vi "CAMERATEST3.vi"() -> ()   [LabVIEW 2016, in "Test2.lvrbt"]
uses:
  Test2.lvrbt
  <vilib>/NXT/Block Support/NXT_InputPort.ctl
  <vilib>/NXT/Subs/ColorSensorColors.ctl
  <vilib>/NXT/Hardware/Plugins/Tetrix DC Motor/TetrixDCMotorAddress.ctl
  <vilib>/NXT/Hardware/Plugins/Tetrix 180 deg Servo/Tetrix180ServoAddress.ctl
  <vilib>/NXT/NXTIO Xnodes/NXTIONodeSubVIs/TETRIX IO Move Servos.vi
  <vilib>/NXT/Dual Mode Library/Waits/Wait_Num.vi
  <vilib>/NXT/NXTIO Xnodes/NXTIONodeSubVIs/TETRIX IO Move DC Motors.vi
  <vilib>/NXT/Dual Mode Library/Waits/Wait_EV3_Color_Color.vi
  <vilib>/NXT/NXTIO Xnodes/NXTIONodeSubVIs/TETRIX IO Stop DC Motors.vi
  <vilib>/NXT/Dual Mode Library/Sound/Tone.vi
  <vilib>/NXT/Dual Mode Library/Sound/StopSound.vi
  <vilib>/NXT/NXTIO Xnodes/AddressXNode/NXTIOAddress.xnode
  <vilib>/NXT/Subs/LVHSConnector.ctl
  <vilib>/NXT/NXTIO Xnodes/NXTIOXNode/NXTIO.xnode
  <vilib>/NXT/LegoClasses/BrickReference/BrickReference.lvclass
panel:
  out "Power":bool
  out "X Upper Left":u8
  out "X Lower Right":u8
  out "Y Lower Right":u8
  out "Y Upper Left":u8
  out "Count":u8
  out "Color":u8
  in  "Cluster":T1 {"Tracking Mode" items=["Disable Tracking", "Get First Object", "Get n th Object", "Enable Tracking", "Sort Objects  by size", "Sort Objects  by Colors", "Illumination on ", "Illumination Off", "Write Colormap", "Read Colormap", "Line tracking mode", "Object Tracking mode"]}
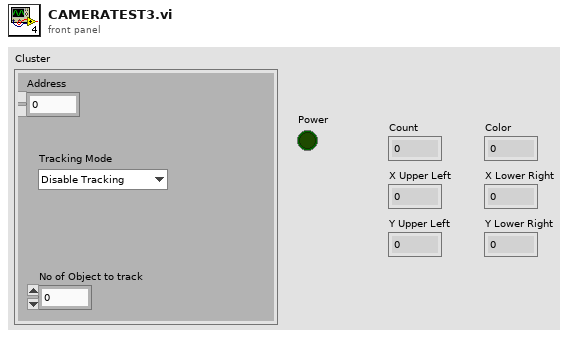
[diagram p1: front panel]
types:
  T1 = cluster{"Address":dbl, "No of Object to track":dbl, "Tracking Mode":u8}
  T2 = typedef "NXT_InputPort.ctl" = u32
  T3 = typedef "ColorSensorColors.ctl" = enum16{"No Color", "Black", "Blue", "Green", "Yellow", "Red", "White", "Brown"}
  T4 = cluster{"Tracking Mode":u8, "Object Number to Track":u8, "Address":u8}
  T5 = typedef "Tetrix180ServoAddress.ctl" = i32
  T6 = cluster{"Tetrix180Servo":T5, "Tetrix180Servo":T5, "Tetrix180Servo":T5, "Tetrix180Servo":T5, "Tetrix180Servo":T5, "Tetrix180Servo":T5}
  T7 = typedef "TetrixDCMotorAddress.ctl" = i32
  T8 = typedef "LVHSConnector.ctl" = refnum<class "BrickReference.lvclass">
  T9 = cluster{"TetrixDCMotor":T7, "TetrixDCMotor 2":T7}
  T10 = cluster{"Total Tracked Objects":u8, "Color":u8, "X Upper Left":u8, "Y Upper Left":u8, "X Lower Right":u8, "Y Lower Right":u8, "Status (boolean)":bool}
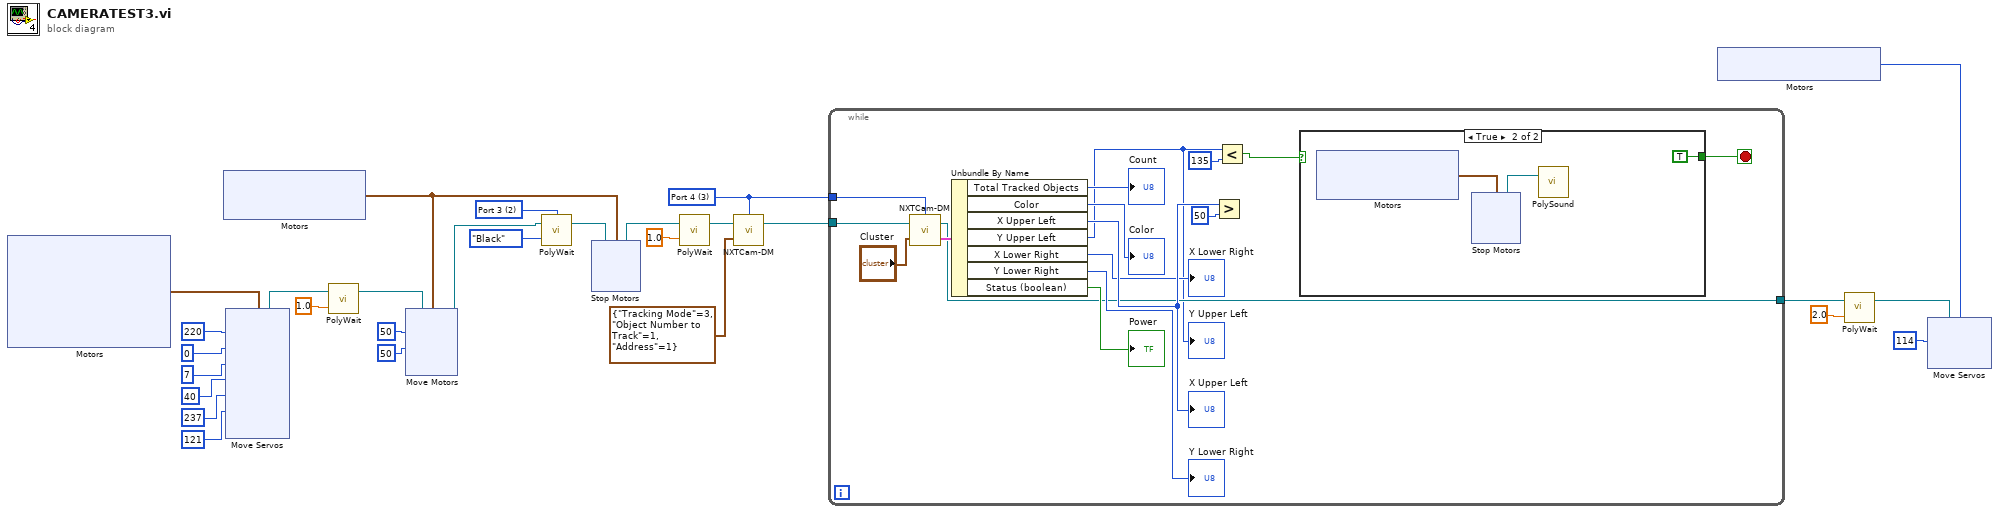
[diagram p0: block diagram]
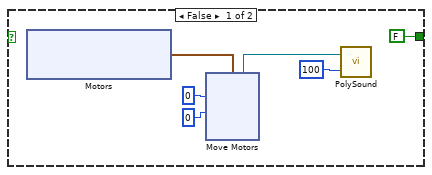
[diagram p2: hidden frame]
diagram:
  w3 = T2 2 items=["Port 1", "Port 2", "Port 3", "Port 4"] ("Port (Port 1)")
  w2 = T2 3 items=["Port 1", "Port 2", "Port 3", "Port 4"] ("Input Port")
  n1 = xnode "Motors"() -> ("Motor"=w16:T6)
  n2 = xnode "Motors"() -> ("Motor"=w25:cluster{"TetrixDCMotor":T7, "TetrixDCMotor":T7})
  n3 = xnode "Move Servos"("Position 6"=u8 121, "Position 5"=u8 237, "Position 4"=u8 40, "Position 3"=u8 7, "Position 2"=u8 0, "Position 1"=u8 220, "Motors"=w16) -> ("NXT/EV3"=w8:T8)  [unwired: 1 in]
  n4 = call-poly <vilib>:"PolyWait.vi"("Time (1 sec)"=sgl 1.0, "NXT/EV3"=w8) -> ("NXT/EV3"=w4:T8)  [unwired: 2 in]
  n5 = xnode "Move Motors"("Power/Speed 2"=i8 50, "Power/Speed 1"=i8 50, "Motors"=w25, "NXT/EV3"=w4) -> ("NXT/EV3"=w6:T8)
  n6 = call-poly <vilib>:"PolyWait.vi"("Color (Red)"=ColorSensorColors."Black", "NXT/EV3"=w6, "Port (Port 1)"=w3) -> ("NXT/EV3"=w5:T8)  [unwired: 1 in]
  n7 = xnode "Stop Motors"("Motors"=w25, "NXT/EV3"=w5) -> ("NXT/EV3"=w24:T8)
  n8 = call-poly <vilib>:"PolyWait.vi"("Time (1 sec)"=sgl 1.0, "NXT/EV3"=w24) -> ("NXT/EV3"=w23:T8)  [unwired: 2 in]
  n9 = call "NXTCam-DM.vi"("Input of NXTCam"=T4 {"Tracking Mode"=3, "Object Number to Track"=1, "Address"=1}, "NXT"=w23, "Input Port"=w2) -> ("NXT dup"=w1:T8)  [unwired: 1 out]
  n10 = while {
    tunnel: w2 -> [w42]
    tunnel: [w33] -> w20
    tunnel: w1 -> [w30]
    stop <- w34 stop-if-true
    n11 = call "NXTCam-DM.vi"("Input of NXTCam"="Cluster", "NXT"=w30, "Input Port"=w42) -> ("Output of NXTCam"=w39:T10, "NXT dup"=w33:T8)
    n12 = Unbundle By Name(w39) -> ("Total Tracked Objects"=→"Count":u8, "Color"=→"Color":u8, "X Upper Left"=w37:u8, "Y Upper Left"=w32:u8, "X Lower Right"=→"X Lower Right":u8, "Y Lower Right"=→"Y Lower Right":u8, "Status (boolean)"=→"Power":bool)
    "X Upper Left" <- w37
    "Y Upper Left" <- w32
    n13 = Greater?(x=w37, y=u8 50) -> ()  [unwired: 1 out]
    n14 = Less?(x=w32, y=u8 135) -> (x < y?=w29:bool)
    n15 = case shown="True" w29 {
      tunnel: [FALSE TRUE] -> w34
      frame False {
        n16 = xnode "Motors"() -> ("Motor"=w50:cluster{"TetrixDCMotor":T7, "TetrixDCMotor":T7})
        n17 = xnode "Move Motors"("Power/Speed 2"=i8 0, "Power/Speed 1"=i8 0, "Motors"=w50) -> ("NXT/EV3"=w46:T8)  [unwired: 1 in]
        n18 = call-poly <vilib>:"PolySound.vi"("Duration (500 ms)"=u16 100, "NXT/EV3"=w46) -> ()  [unwired: 2 in, 1 out]
      }
      frame True {
        n19 = xnode "Motors"() -> ("Motor"=w62:cluster{"TetrixDCMotor":T7, "TetrixDCMotor":T7})
        n20 = xnode "Stop Motors"("Motors"=w62) -> ("NXT/EV3"=w60:T8)  [unwired: 1 in]
        n21 = call-poly <vilib>:"PolySound.vi"("NXT/EV3"=w60) -> ()  [unwired: 3 in, 1 out]
      }
    }
  }
  n22 = xnode "Motors"() -> ("Motor"=w17:T5)
  n23 = call-poly <vilib>:"PolyWait.vi"("Time (1 sec)"=sgl 2.0, "NXT/EV3"=w20) -> ("NXT/EV3"=w19:T8)  [unwired: 2 in]
  n24 = xnode "Move Servos"("Position 1"=u8 114, "Motors"=w17, "NXT/EV3"=w19) -> ()  [unwired: 1 out]
